vi "Set Generation Status.vi"(8 "error in (no error)":errorcluster, 11 "status":T1) -> (0 "error out":errorcluster)   [LabVIEW 2021, in "AnalogGenerationProcess.lvlib"]
uses:
  AnalogGenerationProcess.lvlib
  <vilib>/addons/PointValueMap/PointValueMap.lvlib
  <vilib>/addons/PointValueMap/subVIs/Point_Write_variant.vi
  controls/generation status.ctl
  controls/AudioGenTypeDefs.lvlib
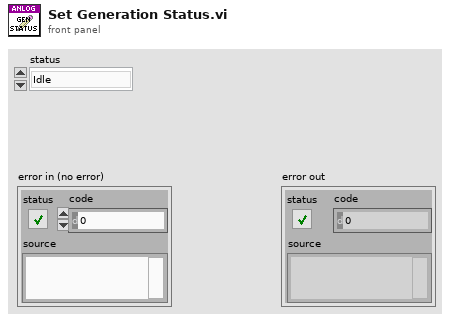
[diagram p1: front panel]
types:
  T1 = typedef "AudioGenTypeDefs.lvlib/generation status.ctl" = enum16{"Idle", "Committed", "Active"}
  T2 = typedef "PointValueMap.lvlib/PointMap.ctl" = refnum<data-value>
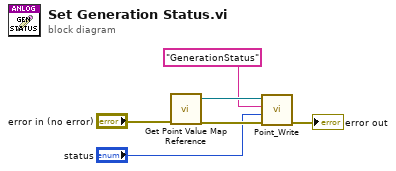
[diagram p0: block diagram]
diagram:
  n1 = call "Get Point Value Map Reference.vi"("error in (no error)"="error in (no error)") -> ("error out"=w5:errorcluster, "Map Out"=w2:T2)  [unwired: 9 in]
  n2 = call-poly <vilib>:"Point_Write.vi"("Error In"=w5, "Value"="status", "Tag"="GenerationStatus", "Map"=w2) -> ("Error Out"=→"error out":errorcluster)  [unwired: 6 in, 1 out]
